vi "AO_WriteRawData16.vi"(4 "error in (no error)":errorcluster, 5 "data":u16[](array[numeric]), 6 "count":i32, 8 "Task ID":u32) -> (0 "error out":errorcluster, 2 "remaining count":i32, 3 "Task ID":u32)   [LabVIEW 2015]
uses:
  Windows/System32/AdvLvDaq.dll
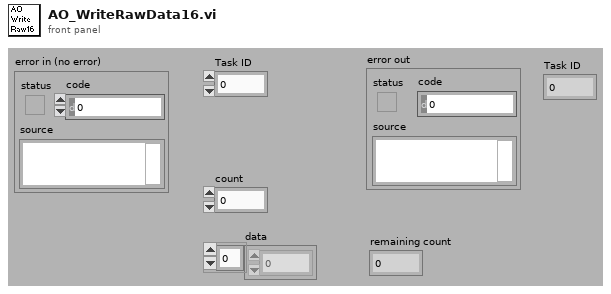
[diagram p1: front panel]
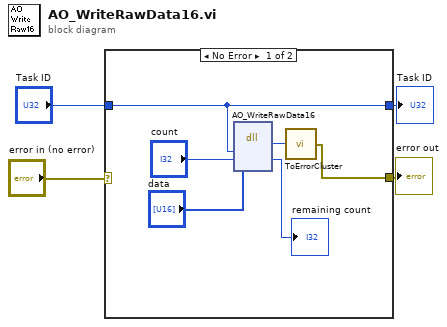
[diagram p0: block diagram]
diagram:
  n1 = case shown="No Error" "error in (no error)" {
    selector: "error in (no error)" -> [_ w12]
    tunnel: [w10 w12] -> w4
    tunnel: "Task ID" -> [w6 w11]
    tunnel: [w6 w11] -> w1
    frame No Error {
      n2 = dll-call lib="C:/Windows/System32/AdvLvDaq.dll" fn="AO_WriteRawData16"("taskId"=w6, "count"="count", "rawData"="data") -> ("return type"=w9:i32, "count"=→"remaining count":i32)  [unwired: 5 in, 2 out]
      n3 = call "ToErrorCluster.vi"("error code"=w9) -> ("error out"=w10:errorcluster)
    }
    frame Error {
    }
  }
  "error out" <- w4
  "Task ID" <- w1
